vi "measure.vi"(8 "error in":errorcluster, 10 "pin map id":string, 11 "measurement configuration":cluster{"Boolean":bool}) -> (0 "error out":errorcluster, 3 "measurement results":cluster{"Boolean":bool})   [LabVIEW 2021, in "Measurement Client Template.lvlib"]
uses:
  Measurement Client Template.lvlib
  <vilib>/gRPC/Generated APIs/ni/measurementlink/discovery/v1/RPC Messages/ni_measurementlink_discovery_v1_ResolveServiceRequest.ctl
  <vilib>/gRPC/Generated APIs/ni/measurementlink/measurement/v2/Measurement Service Client/RPC Messages/ni_measurementlink_measurement_v2_MeasureRequest.ctl
  <vilib>/gRPC/Generated APIs/ni/measurementlink/measurement/v2/Measurement Service Client/RPC Messages/google_protobuf_Any.ctl
  <vilib>/gRPC/Generated APIs/ni/measurementlink/measurement/v2/Measurement Service Client/RPC Messages/ni_measurementlink_PinMapContext.ctl
  17d0f289-ea27-4c60-b0eb-587fd1b50e65.vi
  483b5dc2-6359-43fd-90c2-457bf83eb633.vi
  <vilib>/gRPC/LabVIEW gRPC Library/Server API/Translate Protobuf Error.vi
  <vilib>/AdvancedString/1D String Array to Delimited String.vi
  <vilib>/gRPC/LabVIEW gRPC Library/Server API/Server/Get Server DLL Path.vi
  <vilib>/Plug-In SDKs/Clients/Discovery V1/NI Discovery V1 Client.lvlib
  <vilib>/gRPC/Generated APIs/ni/measurementlink/measurement/v2/Measurement Service Client/Measurement Service Client.lvlib
  <vilib>/gRPC/LabVIEW gRPC Library/grpc-lvsupport-release.lvlib
  <vilib>/gRPC/Generated APIs/ni/measurementlink/discovery/v1/ni.measurementlink.discovery.v1.api.lvlib
panel:
  in  "resolve service request data":T1
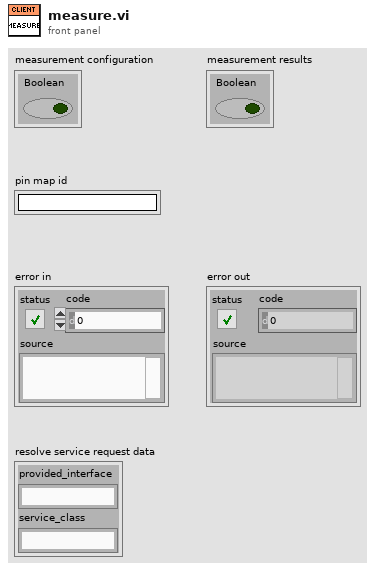
[diagram p1: front panel]
types:
  T1 = typedef "ni.measurementlink.discovery.v1.api.lvlib/ni_measurementlink_discovery_v1_ResolveServiceRequest.ctl" = cluster{"provided_interface":string, "service_class":string}
  T2 = typedef "ni.measurementlink.measurement.v2.api.lvlib/Measurement Service Client.lvlib/ni_measurementlink_measurement_v2_MeasureRequest.ctl" = cluster{"configuration_parameters":T3, "pin_map_context":T4}
  T3 = typedef "ni.measurementlink.measurement.v2.api.lvlib/Measurement Service Client.lvlib/google_protobuf_Any.ctl" = cluster{"type_url":string, "value":u8[]}
  T4 = typedef "ni.measurementlink.measurement.v2.api.lvlib/Measurement Service Client.lvlib/ni_measurementlink_PinMapContext.ctl" = cluster{"pin_map_id":string, "sites":i32[]}
  T5 = typedef "ni.measurementlink.discovery.v1.api.lvlib/ni_measurementlink_discovery_v1_ServiceLocation.ctl" = cluster{"location":string, "insecure_port":string, "ssl_authenticated_port":string}
  T6 = typedef "grpc-lvsupport-release.lvlib/grpcId.ctl" = u64
  T7 = typedef "grpc-lvsupport-release.lvlib/Enum Metadata.ctl" = cluster{"Version":i32, "Name":string, "Type Url":string, "Enum Values":string, "Allow Alias":bool}
  T8 = typedef "grpc-lvsupport-release.lvlib/Message Metadata.ctl" = cluster{"Version":i32, "Name":string, "Type Url":string, "Elements":T9[], "Has Oneof":bool}
  T9 = typedef "grpc-lvsupport-release.lvlib/Message Element Metadata.ctl" = cluster{"Field Name":string, "Embedded Message Name":string, "Protobuf Index":i32, "MessageElementType":T10, "Repeated":bool, "Is in Oneof":bool, "Oneof Container Name":string}
  T10 = typedef "grpc-lvsupport-release.lvlib/Message Element Type.ctl" = enum32{"Int32Value", "FloatValue", "DoubleValue", "BoolValue", "StringValue", "MessageValue", "Int64Value", "UInt32Value", "UInt64Value", "EnumValue", "Bytes", "Fixed64", "Fixed32", "SFixed64", "SFixed32", "SInt64", "SInt32"}
  T11 = typedef "grpc-lvsupport-release.lvlib/Any.ctl" = cluster{"Type Url":string, "Bytes":u8[]}
  T12 = typedef "ni.measurementlink.measurement.v2.api.lvlib/Measurement Service Client.lvlib/ni_measurementlink_measurement_v2_MeasureResponse.ctl" = cluster{"outputs":T3}
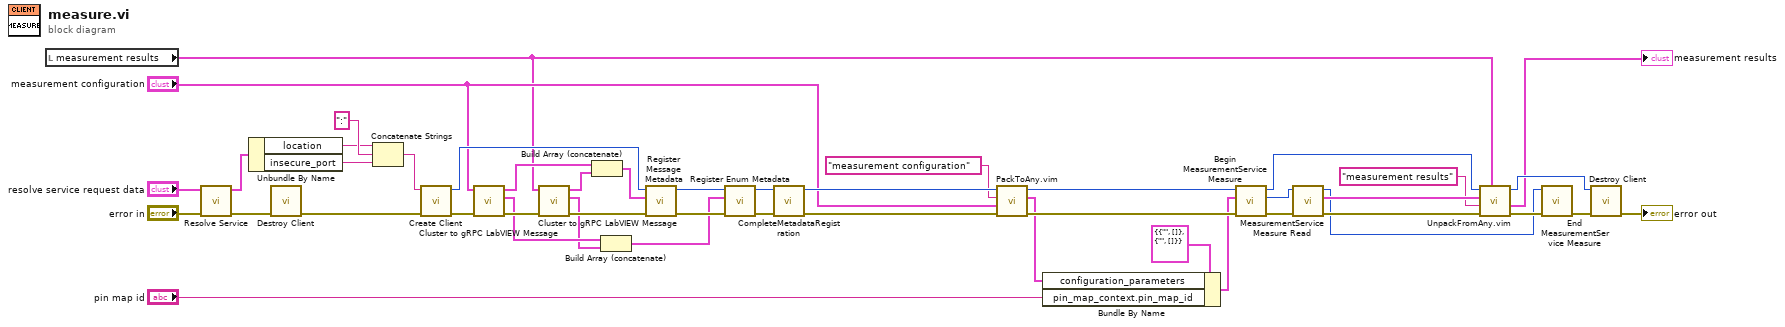
[diagram p0: block diagram]
diagram:
  n1 = local read "measurement results"() -> (w18:cluster{"Boolean":bool})
  n2 = call <vilib>:"Resolve Service.vi"("error in"="error in", "request data"="resolve service request data") -> ("error out"=w44:errorcluster, "response data"=w46:T5)  [unwired: 8 in]
  n3 = Unbundle By Name(w46) -> ("location"=w40:string, "insecure_port"=w41:string)
  n4 = call <vilib>:"Destroy Client.vi"("error in"=w44) -> ("error out"=w42:errorcluster)  [unwired: 10 in]
  n5 = Concatenate Strings(w40, ":" ("string"), w41) -> (w43:string)
  n6 = call <vilib>:"Create Client.vi"("error in"=w42, "address"=w43) -> ("error out"=w37:errorcluster, "gRPC ID Out"=w29:T6)  [unwired: 8 in]
  n7 = call <vilib>:"Cluster to gRPC LabVIEW Message.vi"("error in"=w37, "Cluster"="measurement configuration") -> ("error out"=w38:errorcluster, "gRPC Enum Metadata out"=w2:T7[], "gRPC Message Metadata []"=w30:T8[])  [unwired: 7 in]
  n8 = call <vilib>:"Cluster to gRPC LabVIEW Message.vi"("error in"=w38, "Cluster"=w18) -> ("error out"=w33:errorcluster, "gRPC Enum Metadata out"=w1:T7[], "gRPC Message Metadata []"=w32:T8[])  [unwired: 7 in]
  n9 = Build Array (concatenate)(w30, w32) -> (w31:T8[])
  n10 = Build Array (concatenate)(w2, w1) -> (w3:T7[])
  n11 = call <vilib>:"Register Message Metadata.vi"("error in"=w33, "Messages"=w31, "gRPCid in"=w29) -> ("error out"=w7:errorcluster, "gRPCid out"=w5:T6)  [unwired: 7 in]
  n12 = call <vilib>:"Register Enum Metadata.vi"("error in"=w7, "Enum Metadata"=w3, "gRPCid in"=w5) -> ("error out"=w6:errorcluster, "gRPCid out"=w4:T6)  [unwired: 7 in]
  n13 = call <vilib>:"CompleteMetadataRegistration.vi"("error in"=w6, "gRPC ID in"=w4) -> ("error out"=w34:errorcluster, "gRPC ID Out"=w35:T6)  [unwired: 8 in]
  n14 = call "PackToAny.vim"("error in"=w34, "Data To Pack"="measurement configuration", "Message Type"="measurement configuration", "gRPCid in"=w35) -> ("error out"=w26:errorcluster, "Any"=w25:T11, "gRPCid out"=w9:u64)  [unwired: 5 in]
  n15 = Bundle By Name(cluster=T2 {"configuration_parameters"={"type_url"="", "value"=[]}, "pin_map_context"={"pin_map_id"="", "sites"=[]}} ("Request Data"), "configuration_parameters"=w25, "pin_map_context.pin_map_id"="pin map id") -> (w24:T2)
  n16 = call <vilib>:"Begin MeasurementService Measure.vi"("error in"=w26, "Request Data"=w24, "gRPC ID"=w9) -> ("error out"=w23:errorcluster, "Call Id Out"=w15:T6, "gRPC ID out"=w13:T6)  [unwired: 6 in]
  n17 = call <vilib>:"MeasurementService Measure Read.vi"("error in"=w23, "Call ID in"=w15) -> ("error out"=w22:errorcluster, "Response Data"=w21:T12, "Call ID"=w14:T6)  [unwired: 6 in, 1 out]
  n18 = call "UnpackFromAny.vim"("Data Type"=w18, "error in"=w22, "Message Type"="measurement results", "Any"=w21, "gRPCid in"=w13) -> ("error out"=w17:errorcluster, "Unpacked Value"=→"measurement results":cluster{"Boolean":bool}, "gRPCid out"=w12:u64)  [unwired: 4 in]
  n19 = call <vilib>:"End MeasurementService Measure.vi"("error in"=w17, "Call ID in"=w14) -> ("error out"=w16:errorcluster)  [unwired: 8 in, 1 out]
  n20 = call <vilib>:"Destroy Client.vi"("error in"=w16, "gRPC ID"=w12) -> ("error out"=→"error out":errorcluster)  [unwired: 9 in]
